vi "Intake Manual Control.vi"(8 "Manual In":bool, 9 "Manual Out":bool, 10 "Outtake Speed":dbl, 11 "Intake Speed":dbl) -> (3 "Intake Output":dbl)   [LabVIEW 2017]
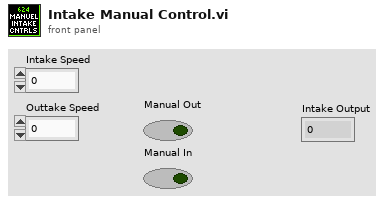
[diagram p1: front panel]
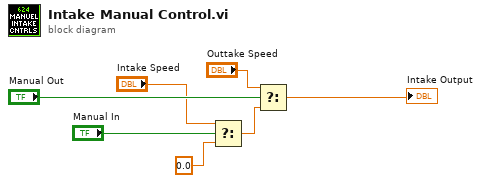
[diagram p0: block diagram]
diagram:
  n1 = Select(t="Intake Speed", s="Manual In", f=0.0) -> (s? t:f=w4:dbl)
  n2 = Select(t="Outtake Speed", s="Manual Out", f=w4) -> (s? t:f=→"Intake Output":dbl)
